vi "Write NET_StreamTask.vi"(8 "error in (no error)":errorcluster, 10 "Task":refnum<k24>, 11 "HttpContent in":refnum<class "HttpContent.lvclass">) -> (0 "error out":errorcluster, 3 "HttpContent out":refnum<class "HttpContent.lvclass">)   [LabVIEW 2018, in "LabVIEWHTTPClient_NET.lvlib" / "HttpContent.lvclass"]
uses:
  HttpContent.lvclass
  HttpContent.lvclass/HttpContent.ctl
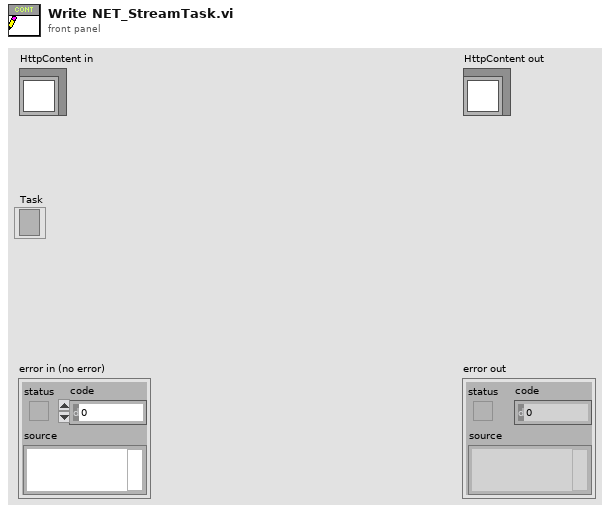
[diagram p1: front panel]
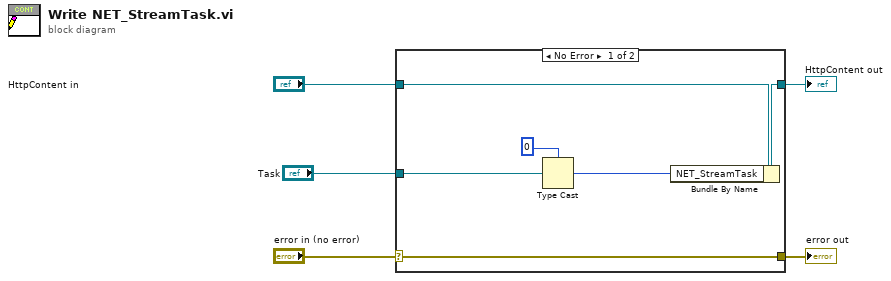
[diagram p0: block diagram]
diagram:
  n1 = case shown="No Error" "error in (no error)" {
    selector: "error in (no error)" -> [w11 w12]
    tunnel: [w11 w12] -> w4
    tunnel: [w9 w13] -> w2
    tunnel: "HttpContent in" -> [w10 w13]
    tunnel: "Task" -> [w8 _]
    frame No Error {
      n2 = Type Cast(type=i64 0 ("NET_StreamTask"), x=w8) -> (*(type *) &x=w7:i64)
      n3 = Bundle By Name(cluster=w10, "NET_StreamTask"=w7) -> (w9:refnum<class "HttpContent.lvclass">)
    }
    frame Error {
    }
  }
  "error out" <- w4
  "HttpContent out" <- w2
